vi "New Null Buffer.vi"(7 "byte order (host order)":T1(ring)=enum."native, host order", 8 "error in (no error)":errorcluster, 9 "buffer offset":u64 format="%d bytes", 10 "buffer size":u64 format="%d bytes", 11 "Buffer type":refnum<class "Buffer.lvclass">) -> (0 "error out":errorcluster, 3 "Buffer out":refnum<class "Buffer.lvclass">)   [LabVIEW 2017, in "DSF Core.lvlib" / "Buffer.lvclass"]
doc: "Creates a new, unallocated, Buffer object."
uses:
  Buffer.lvclass
  C:/Git/DSF/LabVIEW-Memory/Source/Classes/Pointer/Pointer.lvclass
  Buffer.lvclass/Buffer.ctl
  LabVIEW-Memory/Source/Classes/Pointer/Pointer.lvclass
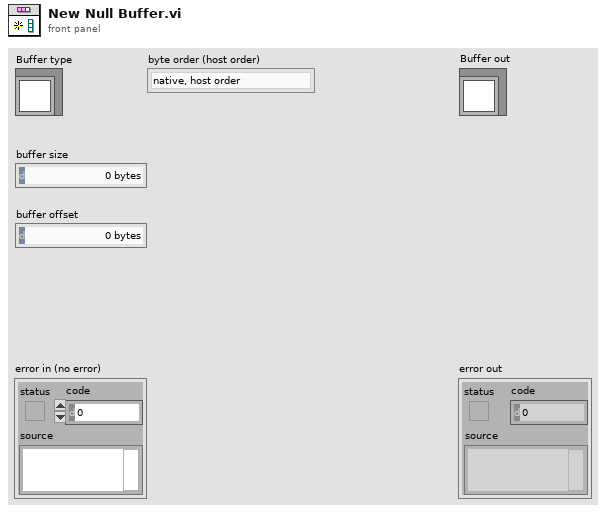
[diagram p1: front panel]
types:
  T1 = enum16{"big-endian, network order", "native, host order", "little-endian"}
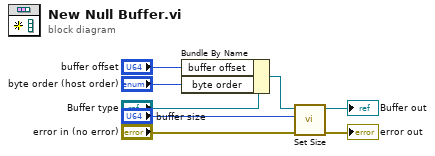
[diagram p0: block diagram]
diagram:
  n1 = Bundle By Name(cluster="Buffer type", "buffer offset"="buffer offset", "byte order"="byte order (host order)") -> (w3:refnum<class "Buffer.lvclass">)
  n2 = call "Set Size.vi"("size"="buffer size", "Pointer in"=w3) -> ("Pointer out"=→"Buffer out":refnum<class "Buffer.lvclass">)  [unwired: 9 in]
  "error out" <- "error in (no error)"
